vi "Create.vi"(7 "buffer size (10)":i32=10, 8 "error in (no error)":errorcluster, 10 "Ctrl Val.Set All":T2[](array[typedef]), 11 "name (unnamed)":string) -> (0 "error out":errorcluster, 3 "All Queue out":T1)   [LabVIEW 2015, in "UndoLibrary.lvlib"]
doc: "This VI creates the references to store the values of the controls.\n\n- x.current: Contains the current value of the controls. (Size: 1).\n- x.undo: Allows to store the changes in the controls. (Size: Buffer).\n- x.redo: Allows to store the changes in the controls. (Size: Buffer)."
uses:
  UndoLibrary.lvlib
  Controls/cluster_Control Value.ctl
  Controls/cluster_All Queue.ctl
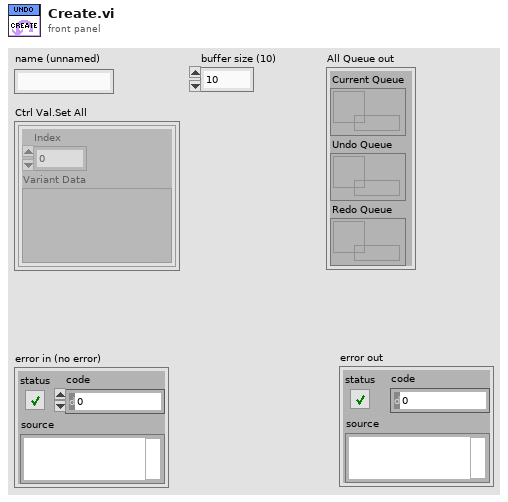
[diagram p1: front panel]
types:
  T1 = typedef "UndoLibrary.lvlib/cluster_All Queue.ctl" = cluster{"Current Queue":refnum<queue>, "Undo Queue":refnum<queue>, "Redo Queue":refnum<queue>}
  T2 = typedef "UndoLibrary.lvlib/cluster_Control Value.ctl" = cluster{"Index":i32, "Variant Data":variant}
  T3 = cluster{"queue out":refnum<queue>, "queue out":refnum<queue>, "queue out":refnum<queue>}
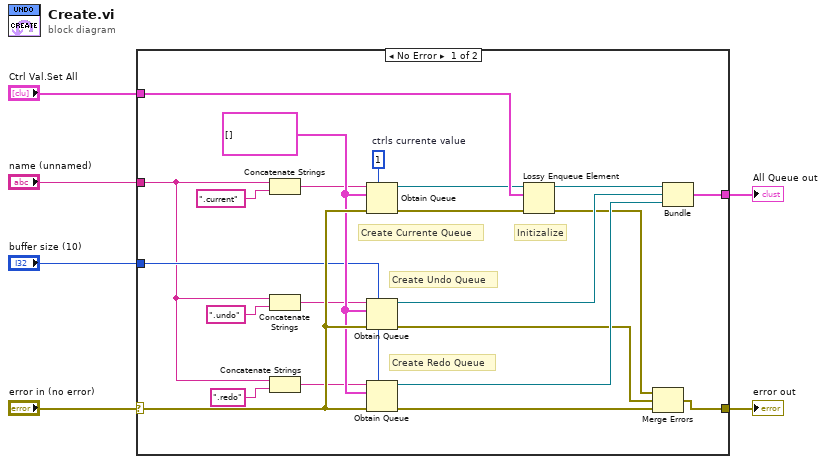
[diagram p0: block diagram]
diagram:
  n1 = case shown="No Error" "error in (no error)" {
    selector: "error in (no error)" -> [w25 w29]
    tunnel: "Ctrl Val.Set All" -> [w28 _]
    tunnel: "buffer size (10)" -> [w22 _]
    tunnel: "name (unnamed)" -> [w20 _]
    tunnel: [w10 _] -> w2
    tunnel: [w9 w29] -> w1
    frame No Error {
      w23 = 1  # ctrls currente value
      w24 = T2[] []
      # "Create Redo Queue"
      # "Create Undo Queue"
      # "Initizalize"
      # "Create Currente Queue"
      n2 = Concatenate Strings(w20, ".current" ("name (unnamed)")) -> (w16:string)
      n3 = Concatenate Strings(w20, ".undo" ("name (unnamed)")) -> (w15:string)
      n4 = Concatenate Strings(w20, ".redo" ("name (unnamed)")) -> (w14:string)
      n5 = Obtain Queue(max queue size (-1, unlimited)=w23, name (unnamed)=w16, element data type=w24, error in (no error)=w25) -> (queue out=w26:refnum<queue>, error out=w27:errorcluster)  [unwired: 1 in, 1 out]
      n6 = Obtain Queue(max queue size (-1, unlimited)=w22, name (unnamed)=w15, element data type=w24, error in (no error)=w25) -> (queue out=w12:refnum<queue>, error out=w7:errorcluster)  [unwired: 1 in, 1 out]
      n7 = Obtain Queue(max queue size (-1, unlimited)=w22, name (unnamed)=w14, element data type=w24, error in (no error)=w25) -> (queue out=w11:refnum<queue>, error out=w21:errorcluster)  [unwired: 1 in, 1 out]
      n8 = Lossy Enqueue Element(queue=w26, element=w28, error in (no error)=w27) -> (queue out=w13:refnum<queue>, error out=w8:errorcluster)  [unwired: 2 out]
      n9 = Merge Errors(w8, w7, w21) -> (w9:errorcluster)
      n10 = Bundle("queue out"=w13, "queue out"=w12, "queue out"=w11) -> (w10:T3)  [unwired: 1 in]
    }
    frame Error {
    }
  }
  "error out" <- w1
  "All Queue out" <- w2
